vi "cyclic_receiver.vi"(0 "IQ Rate [S/sec]":dbl=2000000.0 format="%#_6p", 1 "pulse duration[sample]":i32=5, 2 "level":dbl=0.01 format="%#_13g", 4 "M":i8=16, 5 "reference":refnum<vi>, 6 "Symbol per cycle":i32=100, 13 "simboli da ricevere":i32=101250) -> (14 "received symbols":i8[](array[numeric]), 16 "first sample found":bool=TRUE, 17 "synchro sequence found":bool)   [LabVIEW 2017]
uses:
  <instrlib>/niUSRP/niUSRP Fetch Rx Data (CDB).vi
panel:
  out "Numeric 2":i32
  in  "Synchro":i8[](array[numeric])=[0, 1, 1, 0, 1, 0, 0, 0, 0, 0, 0, 0, 1, 0, 0, 0, 0, 0, 1, 1]
  out "Numeric":i32
  out "size(s)":i32
  out "end found":bool=TRUE
  out "BIT RICEVUTI":i32=40000
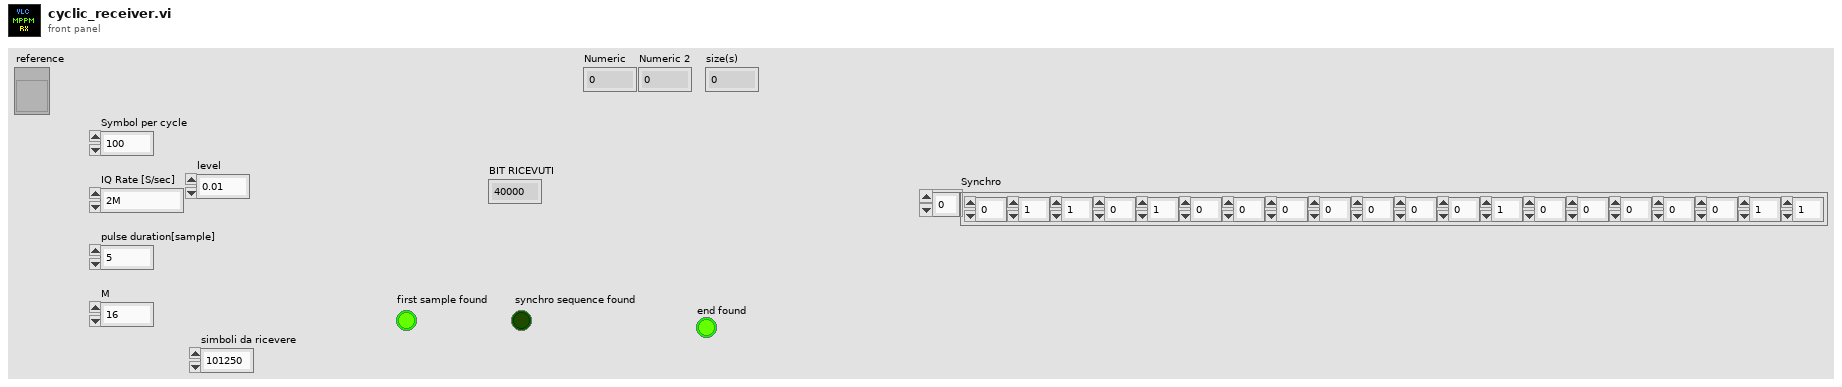
[diagram p1: front panel]
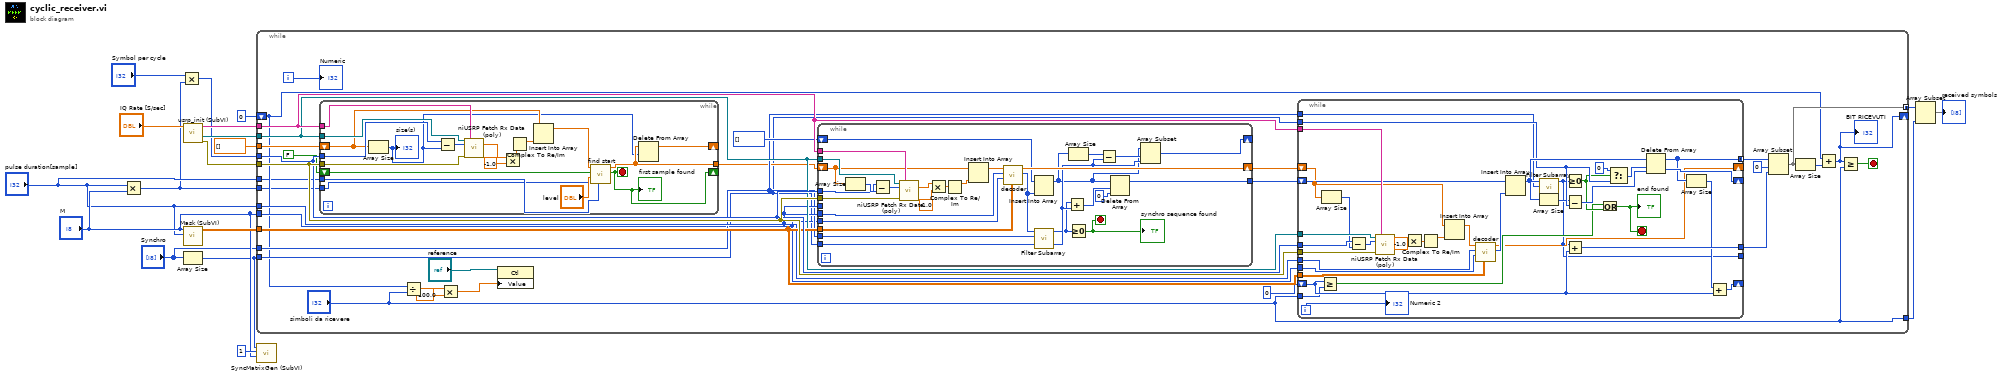
[diagram p0: block diagram]
diagram:
  n1 = Multiply(x="pulse duration[sample]", y="M") -> (x*y=w1:i32)
  n2 = Multiply(x="Symbol per cycle", y=w1) -> (x*y=w5:i32)
  n3 = call "usrp_init (SubVI).vi"("IQ Rate [S/sec]"="IQ Rate [S/sec]") -> ("error out"=w18:errorcluster, "IVI Refnum out"=w15:refnum<k15>, "Enabled Channel out"=w16:string)  [unwired: 7 in]
  n4 = call "Mask (SubVI).vi"("pulse duration[sample]"="pulse duration[sample]", "M"="M") -> ("Array"=w17:dbl[][])  [unwired: 9 in]
  n5 = Array Size(array="Synchro") -> (size(s)=w3:i32)
  n6 = while {
    tunnel: w18 -> [w50]
    tunnel: w5 -> [w49]
    tunnel: w17 -> [w48]
    tunnel: w16 -> [w47]
    tunnel: w15 -> [w46]
    tunnel: "pulse duration[sample]" -> [w42]
    tunnel: w3 -> [w29]
    tunnel: "Synchro" -> [w41]
    tunnel: "M" -> [w40]
    tunnel: [w37] -> w10 mode=concatenating
    shift-right: [w27] -> _
    shift-left: 0 -> [w24]
    tunnel: ["simboli da ricevere"] -> w11
    tunnel: dbl[] [] ("signal out") -> [w30]
    tunnel: "pulse duration[sample]" -> [w20]
    tunnel: w1 -> [w19]
    i -> [w28]
    stop <- w35 stop-if-true
    n7 = while {
      shift-right: [w131] -> _
      shift-left: FALSE ("Trigger found") -> [w135]
      tunnel: w47 -> [w134]
      tunnel: w50 -> [w133]
      tunnel: w46 -> [w132]
      tunnel: w49 -> [w126]
      shift-right: [w128] -> _
      shift-left: w30 -> [w125]
      tunnel: [w129] -> w39
      tunnel: w20 -> [w121]
      tunnel: w19 -> [w120]
      stop <- w131 stop-if-true
      n8 = Array Size(array=w125) -> (size(s)=w122:i32)
      "size(s)" <- w122
      n9 = Subtract(x=w126, y=w122) -> (x-y=w124:i32)
      n10 = call-poly <instrlib>:"niUSRP Fetch Rx Data (poly).vi"("session handle"=w132, "channel list"=w134, "number of samples"=w124, "error in (no error)"=w133) -> ("data"=w118:cdb[])  [unwired: 8 in, 3 out]
      n11 = Multiply(x=w118, y=-1.0) -> (x*y=w117:cdb[])
      n12 = Complex To Re/Im(x + iy=w117) -> (x=w127:dbl[])  [unwired: 1 out]
      n13 = Insert Into Array(array=w125, new element=w127) -> (w123:dbl[])  [unwired: 1 in]
      n14 = call "find start.vi"("pulse sample"=w121, "trama length"=w120, "level"="level", "Trigger found in"=w135, "signal in"=w123) -> ("Trigger found"=w131:bool, "signal out"=w129:dbl[])  [unwired: 5 in]
      "first sample found" <- w131
      n15 = Delete From Array(array=w129, length=w122) -> (array with subset deleted=w128:dbl[])  [unwired: 1 in, 1 out]
    }
    n16 = Divide(x=w24, y="simboli da ricevere") -> (x/y=w23:dbl)
    n17 = Multiply(x=w23, y=100.0) -> (x*y=w22:dbl)
    n18 = property class="Ctl"(reference="reference", "Value"=w22) -> ()  [unwired: 1 in, 2 out]
    n19 = while {
      tunnel: w46 -> [w116]
      tunnel: w47 -> [w115]
      tunnel: w50 -> [w114]
      shift-right: [w108] -> w45
      shift-left: w39 -> [w96]
      shift-right: [w104] -> _
      shift-left: i32[] [] ("array") -> [w100]
      tunnel: w48 -> [w112]
      tunnel: w40 -> [w111]
      tunnel: w42 -> [w110]
      tunnel: w49 -> [w94]
      tunnel: w41 -> [w109]
      tunnel: w42 -> [_]
      tunnel: w29 -> [w102]
      tunnel: [w105] -> w34
      stop <- w91 stop-if-true
      n20 = Array Size(array=w96) -> (size(s)=w95:i32)
      n21 = Subtract(x=w94, y=w95) -> (x-y=w93:i32)
      n22 = call-poly <instrlib>:"niUSRP Fetch Rx Data (poly).vi"("session handle"=w116, "channel list"=w115, "number of samples"=w93, "error in (no error)"=w114) -> ("data"=w89:cdb[])  [unwired: 8 in, 3 out]
      n23 = Multiply(x=w89, y=-1.0) -> (x*y=w88:cdb[])
      n24 = Complex To Re/Im(x + iy=w88) -> (x=w97:dbl[])  [unwired: 1 out]
      n25 = Insert Into Array(array=w96, new element=w97) -> (w113:dbl[])  [unwired: 1 in]
      n26 = call "decoder.vi"("Mask"=w112, "M"=w111, "pulse duration[sample]"=w110, "input signal"=w113) -> ("Array out"=w99:i32[], "residual samples"=w108:dbl[])  [unwired: 6 in]
      n27 = Insert Into Array(array=w100, new element=w99) -> (w98:i32[])  [unwired: 1 in]
      n28 = call "Filter Subarray.vi"("Subarray"=w109, "Array"=w99) -> ("Index of Subarray"=w92:i32)  [unwired: 9 in]
      n29 = Add(x=w92, y=w102) -> (x+y=w106:i32)
      n30 = Array Size(array=w98) -> (size(s)=w103:i32)
      n31 = Greater Or Equal To 0?(x=w92) -> (x >= 0?=w91:bool)
      "synchro sequence found" <- w91
      n32 = Subtract(x=w103, y=w102) -> (x-y=w101:i32)
      n33 = Delete From Array(array=w98, length=w106, index=0) -> (array with subset deleted=w105:i32[])  [unwired: 1 out]
      n34 = Array Subset(array=w98, index=w101, length=w102) -> (w104:i32[])
    }
    n35 = while {
      shift-right: [w57] -> _
      shift-left: w45 -> [w60]
      tunnel: [w70] -> w33 mode=concatenating
      tunnel: w46 -> [w87]
      tunnel: w47 -> [w86]
      tunnel: w48 -> [w85]
      tunnel: w40 -> [w84]
      tunnel: w49 -> [w62]
      tunnel: "simboli da ricevere" -> [w67]
      tunnel: w50 -> [w83]
      tunnel: w42 -> [w82]
      tunnel: w41 -> [w55]
      shift-right: [w81] -> _
      shift-left: w34 -> [w79]
      tunnel: w29 -> [w76]
      shift-right: [w72] -> _
      shift-left: 0 -> [w68]
      tunnel: [w71] -> w31
      tunnel: [w56] -> _
      i -> [w54]
      stop <- w66 stop-if-true
      n36 = Greater Or Equal?(x=w68, y=w67) -> (x >= y?=w64:bool)
      n37 = Array Size(array=w60) -> (size(s)=w59:i32)
      n38 = Subtract(x=w62, y=w59) -> (x-y=w61:i32)
      n39 = call-poly <instrlib>:"niUSRP Fetch Rx Data (poly).vi"("session handle"=w87, "channel list"=w86, "number of samples"=w61, "error in (no error)"=w83) -> ("data"=w51:cdb[])  [unwired: 8 in, 3 out]
      n40 = Multiply(x=w51, y=-1.0) -> (x*y=w53:cdb[])
      n41 = Complex To Re/Im(x + iy=w53) -> (x=w63:dbl[])  [unwired: 1 out]
      n42 = Insert Into Array(array=w60, new element=w63) -> (w58:dbl[])  [unwired: 1 in]
      n43 = call "decoder.vi"("Mask"=w85, "M"=w84, "pulse duration[sample]"=w82, "input signal"=w58) -> ("Array out"=w78:i32[], "residual samples"=w57:dbl[])  [unwired: 6 in]
      n44 = Insert Into Array(array=w79, new element=w78) -> (w77:i32[])  [unwired: 1 in]
      n45 = call "Filter Subarray.vi"("Subarray"=w55, "Array"=w77) -> ("Index of Subarray"=w56:i32)  [unwired: 9 in]
      n46 = Array Size(array=w77) -> (size(s)=w73:i32)
      n47 = Greater Or Equal To 0?(x=w56) -> (x >= 0?=w65:bool)
      n48 = Subtract(x=w73, y=w76) -> (x-y=w80:i32)
      n49 = Add(x=w56, y=w68) -> (x+y=w71:i32)
      n50 = Or(x=w64, y=w65) -> (x .or. y?=w66:bool)
      "end found" <- w66
      n51 = Select(t=0, s=w65, f=w76) -> (s? t:f=w74:i32)
      n52 = Delete From Array(array=w77, length=w74, index=w80) -> (deleted portion=w81:i32[], array with subset deleted=w70:i32[])
      n53 = Array Size(array=w70) -> (size(s)=w69:i32)
      n54 = Add(x=w69, y=w68) -> (x+y=w72:i32)
      "Numeric 2" <- w54
    }
    n55 = Array Subset(array=w33, index=0, length=w31) -> (w37:i32[])
    n56 = Array Size(array=w37) -> (size(s)=w36:i32)
    n57 = Add(x=w24, y=w36) -> (x+y=w27:i32)
    "BIT RICEVUTI" <- w27
    n58 = Greater Or Equal?(x=w27, y="simboli da ricevere") -> (x >= y?=w35:bool)
    "Numeric" <- w28
  }
  n59 = call "SyncMatrixGen (SubVI).vi"("M"="M", "Hamming distance"=1, "Length"=w3) -> ()  [unwired: 8 in, 1 out]
  n60 = Array Subset(array=w10, length=w11) -> (→"received symbols":i32[])  [unwired: 1 in]
